vi "svx_Timebase Exec Commands.vi"(5 "Display State In":T2={"X Scale"={"Name"="Time", "FString"="%#.2g", "Major Color"=16777238, "Minor Color"=16777216, "Grid Style"=1, "Maximum"=0.5, "Minimum"=0.0, "Autoscale"=TRUE, "Show Scale Label"={"Probe X"=FALSE, "Probe Y"=TRUE}, "Show Scale"={"Probe X"=TRUE, "Probe Y"=TRUE}, "Autoscale Once"=FALSE}, "Y Scale"={"Name"="Amplitude", "FString"="%#.2g", "Major Color"=16777238, "Minor Color"=16777216, "Scale Visible"=TRUE, " Label Visible"=TRUE, "Grid Style"=1, "Autoscale"=TRUE, "Maximum"={"Probe X"=1.0, "Probe Y"=1.0}, "Minimum"={"Probe X"=-1.0, "Probe Y"=-1.0}, "Autoscale Once"=FALSE}, "Plot"={"Point Style"=0, "Line Width"=0, "Line Style"=0, "Plot Color"=16860, "Point/fill"=16860}, "Tacho Point Color"=16711680, "Property Name"=[], "Container Bounds"={"Width"=640, "Height"=360}, "Background color"=16777226, "Legend Visible"=TRUE, "Scale Range Change"=refnum, "Strings[]"={"Custom pair name"=FALSE, "Row Strings []"=[], "Column Strings []"=[]}, "Cursor"={"Cursor Point Style"=13, "Cursor Style"=5, "Cursor Line Width"=1, "Cursor Line Style"=0, "Cursor Color"=16860, "Cursor Name Visible"=TRUE, "Cursor Visible"=TRUE, "Cursor Lock"=FALSE, "Cursor Index"=0}, "Index"=[], "Legend Width"=200, " Parents Tags"=[], "Children Tags"=[], "Open?"=[], "Label"="Timebase Plot", "Cursor X Pos"={"X"=0.0, "Y"=0.0}, "Cursor Y Pos"={"X"=0.0, "Y"=0.0}, "Graph Type"=enum."Probe X and Y", "Prev Graph Type"=enum."Probe X and Y", "Prev Legend Visible"=TRUE, "Cursor Release"=refnum, "Pair Strings Changed?"=FALSE, "Cursor ID"=refnum, "Legend Background"=16777226, "Legend Font"=16777222, "Probe Y Label"="Probe Y", "Probe X Label"="Probe X", "Probe X Label Visible"=TRUE, "Probe Y Label Visible"=TRUE, "Tree Item Width"=200, "# Custom RowStr"=0, "# Custom ColStr"=0, "Property Name"=refnum, "Data Related State"=refnum} caption="State", 7 "Data In":T7, 8 "Commands":T6[](array[typedef]), 9 "Facade VI":refnum<vi>, 10 "Ref Ins":T1, 11 "Container":refnum<vi>) -> (3 "Display State Out":T2={"X Scale"={"Name"="Time", "FString"="%#.2g", "Major Color"=16777238, "Minor Color"=16777216, "Grid Style"=1, "Maximum"=0.5, "Minimum"=0.0, "Autoscale"=TRUE, "Show Scale Label"={"Probe X"=FALSE, "Probe Y"=TRUE}, "Show Scale"={"Probe X"=TRUE, "Probe Y"=TRUE}, "Autoscale Once"=FALSE}, "Y Scale"={"Name"="Amplitude", "FString"="%#.2g", "Major Color"=16777238, "Minor Color"=16777216, "Scale Visible"=TRUE, " Label Visible"=TRUE, "Grid Style"=1, "Autoscale"=TRUE, "Maximum"={"Probe X"=1.0, "Probe Y"=1.0}, "Minimum"={"Probe X"=-1.0, "Probe Y"=-1.0}, "Autoscale Once"=FALSE}, "Plot"={"Point Style"=0, "Line Width"=0, "Line Style"=0, "Plot Color"=16860, "Point/fill"=16860}, "Tacho Point Color"=16711680, "Property Name"=[], "Container Bounds"={"Width"=640, "Height"=360}, "Background color"=16777226, "Legend Visible"=TRUE, "Scale Range Change"=refnum, "Strings[]"={"Custom pair name"=FALSE, "Row Strings []"=[], "Column Strings []"=[]}, "Cursor"={"Cursor Point Style"=13, "Cursor Style"=5, "Cursor Line Width"=1, "Cursor Line Style"=0, "Cursor Color"=16860, "Cursor Name Visible"=TRUE, "Cursor Visible"=TRUE, "Cursor Lock"=FALSE, "Cursor Index"=0}, "Index"=[], "Legend Width"=200, " Parents Tags"=[], "Children Tags"=[], "Open?"=[], "Label"="Timebase Plot", "Cursor X Pos"={"X"=0.0, "Y"=0.0}, "Cursor Y Pos"={"X"=0.0, "Y"=0.0}, "Graph Type"=enum."Probe X and Y", "Prev Graph Type"=enum."Probe X and Y", "Prev Legend Visible"=TRUE, "Cursor Release"=refnum, "Pair Strings Changed?"=FALSE, "Cursor ID"=refnum, "Legend Background"=16777226, "Legend Font"=16777222, "Probe Y Label"="Probe Y", "Probe X Label"="Probe X", "Probe X Label Visible"=TRUE, "Probe Y Label Visible"=TRUE, "Tree Item Width"=200, "# Custom RowStr"=0, "# Custom ColStr"=0, "Property Name"=refnum, "Data Related State"=refnum} caption="State")   [LabVIEW 2017, in "SVX Timebase.xctl"]
uses:
  <vilib>/addons/_XControls/Timebase Plot/SVX Timebase.xctl
  <vilib>/addons/_XControls/Timebase Plot/subVIs/svx_Timebase Data.ctl
  <vilib>/addons/_XControls/Timebase Plot/subVIs/svx_Timebase State.ctl
  <vilib>/addons/_XControls/Timebase Plot/subVIs/svx_Timebase Bounds.ctl
  <vilib>/addons/_XControls/Timebase Plot/subVIs/svx_Timebase Graph Types.ctl
  <vilib>/addons/_XControls/Timebase Plot/subVIs/svx_Timebase Data Related State.ctl
  <vilib>/addons/_XControls/Timebase Plot/subVIs/svx_Timebase Core States.ctl
panel:
  out "error out":errorcluster
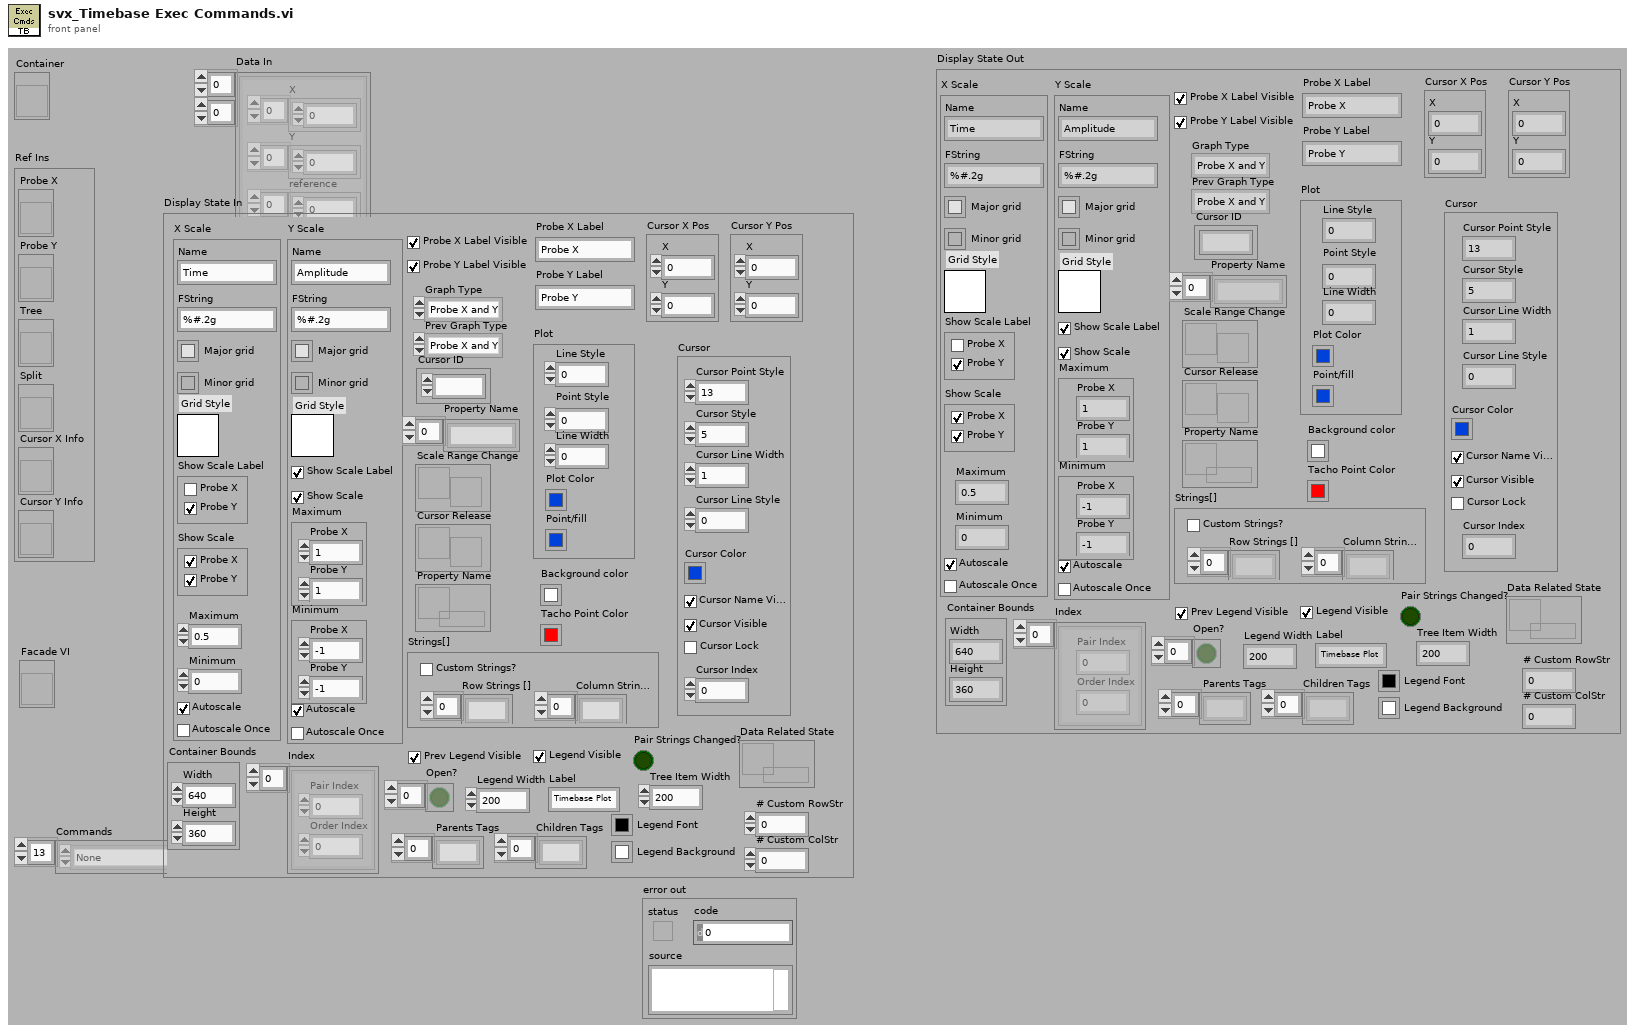
[diagram p1: front panel]
types:
  T1 = cluster{"Probe X":refnum<vi>, "Probe Y":refnum<vi>, "Tree":refnum<vi>, "Split":refnum<vi>, "Cursor X Info":refnum<vi>, "Cursor Y Info":refnum<vi>}
  T2 = typedef "SVX Timebase.xctl/svx_Timebase State.ctl" = cluster{"X Scale":cluster{"Name":string, "FString":string, "Major Color":u32, "Minor Color":u32, "Grid Style":u16, "Maximum":dbl, "Minimum":dbl, "Autoscale":bool, "Show Scale Label":cluster{"Probe X":bool, "Probe Y":bool}, "Show Scale":cluster{"Probe X":bool, "Probe Y":bool}, "Autoscale Once":bool}, "Y Scale":cluster{"Name":string, "FString":string, "Major Color":u32, "Minor Color":u32, "Scale Visible":bool, " Label Visible":bool, "Grid Style":u16, "Autoscale":bool, "Maximum":cluster{"Probe X":dbl, "Probe Y":dbl}, "Minimum":cluster{"Probe X":dbl, "Probe Y":dbl}, "Autoscale Once":bool}, "Plot":cluster{"Point Style":u8, "Line Width":u8, "Line Style":u8, "Plot Color":u32, "Point/fill":u32}, "Tacho Point Color":u32, "Property Name":string[], "Container Bounds":T3, "Background color":u32, "Legend Visible":bool, "Scale Range Change":refnum<user-event>, "Strings[]":cluster{"Custom pair name":bool, "Row Strings []":string[], "Column Strings []":string[]}, "Cursor":cluster{"Cursor Point Style":u8, "Cursor Style":u8, "Cursor Line Width":u8, "Cursor Line Style":u8, "Cursor Color":u32, "Cursor Name Visible":bool, "Cursor Visible":bool, "Cursor Lock":bool, "Cursor Index":i32}, "Index":cluster{"Pair Index":u32, "Order Index":u32}[], "Legend Width":u32, " Parents Tags":string[], "Children Tags":string[], "Open?":bool[], "Label":string, "Cursor X Pos":cluster{"X":dbl, "Y":dbl}, "Cursor Y Pos":cluster{"X":dbl, "Y":dbl}, "Graph Type":T4, "Prev Graph Type":T4, "Prev Legend Visible":bool, "Cursor Release":refnum<user-event>, "Pair Strings Changed?":bool, "Cursor ID":refnum<k1>, "Legend Background":u32, "Legend Font":u32, "Probe Y Label":string, "Probe X Label":string, "Probe X Label Visible":bool, "Probe Y Label Visible":bool, "Tree Item Width":u32, "# Custom RowStr":u32, "# Custom ColStr":u32, "Property Name":refnum<queue>, "Data Related State":T5}
  T3 = typedef "SVX Timebase.xctl/svx_Timebase Bounds.ctl" = cluster{"Width":u32, "Height":u32}
  T4 = typedef "SVX Timebase.xctl/svx_Timebase Graph Types.ctl" = enum16{"Probe X", "Probe Y", "Probe X and Y"}
  T5 = typedef "SVX Timebase.xctl/svx_Timebase Data Related State.ctl" = refnum<queue>
  T6 = typedef "SVX Timebase.xctl/svx_Timebase Core States.ctl" = enum16{"None", "[Axis] Range X Scale", "[Axis] Range Y Scale", "[Layout] Graph Type Change", "[Plot] Tacho Point", "[Plot] Grid and BG", "[Cursor] Cursor Info", "[Legend] Pair Strings", "[Data] Plot Data", "[Legend] Checkbox", "[Layout] Update", "[Legend] Tree Open", "[Layout] Legend Visible Change", "[Plot] Data Point", "[Cursor] Appearance", "[Cursor] Index", "[Legend] Color", "[Axis] Axis and Label", "[Axis] Format String", "[Layout] Min Pane Size", "[Data] Index", "[Plot] Caption", "[Data] Legend Strings"}
  T7 = typedef "SVX Timebase.xctl/svx_Timebase Data.ctl" = cluster{"X":dbl[], "Y":dbl[], "reference":dbl[], "plot type":enum16{"Filtered Plot", "Unfiltered Plot"}, "attribute":variant}[][]
  T8 = cluster{"Queue Newer?":bool, "State Newer?":bool, "Maximum":dbl, "Minimum":dbl, "Maximum":cluster{"Probe X":dbl, "Probe Y":dbl}, "Minimum":cluster{"Probe X":dbl, "Probe Y":dbl}, "Cursor Index":i32, "Cursor X Pos":cluster{"X":dbl, "Y":dbl}, "Cursor Y Pos":cluster{"X":dbl, "Y":dbl}, "Strings[]":cluster{"Custom pair name":bool, "Row Strings []":string[], "Column Strings []":string[]}, "Index":cluster{"Pair Index":u32, "Order Index":u32}[], "Tree Item Width":u32, "Parents Tags":string[], "Children Tags":string[], "Open?":bool[], "Tree Visible?":bool, "Graph Type":T4, "Container Bounds":T3, "Label":string}
  T9 = cluster{"X":dbl[], "Y":dbl[], "reference":dbl[], "plot type":enum16{"Filtered Plot", "Unfiltered Plot"}, "attribute":variant}
  T10 = cluster{"Cursor Point Style":u8, "Cursor Style":u8, "Cursor Line Width":u8, "Cursor Line Style":u8, "Cursor Color":u32, "Cursor Name Visible":bool, "Cursor Visible":bool, "Cursor Lock":bool, "Cursor Index":i32}
  T11 = typedef "LVPointDoubleTypeDef.ctl" = cluster{"Cursor X":dbl, "Cursor Y":dbl}
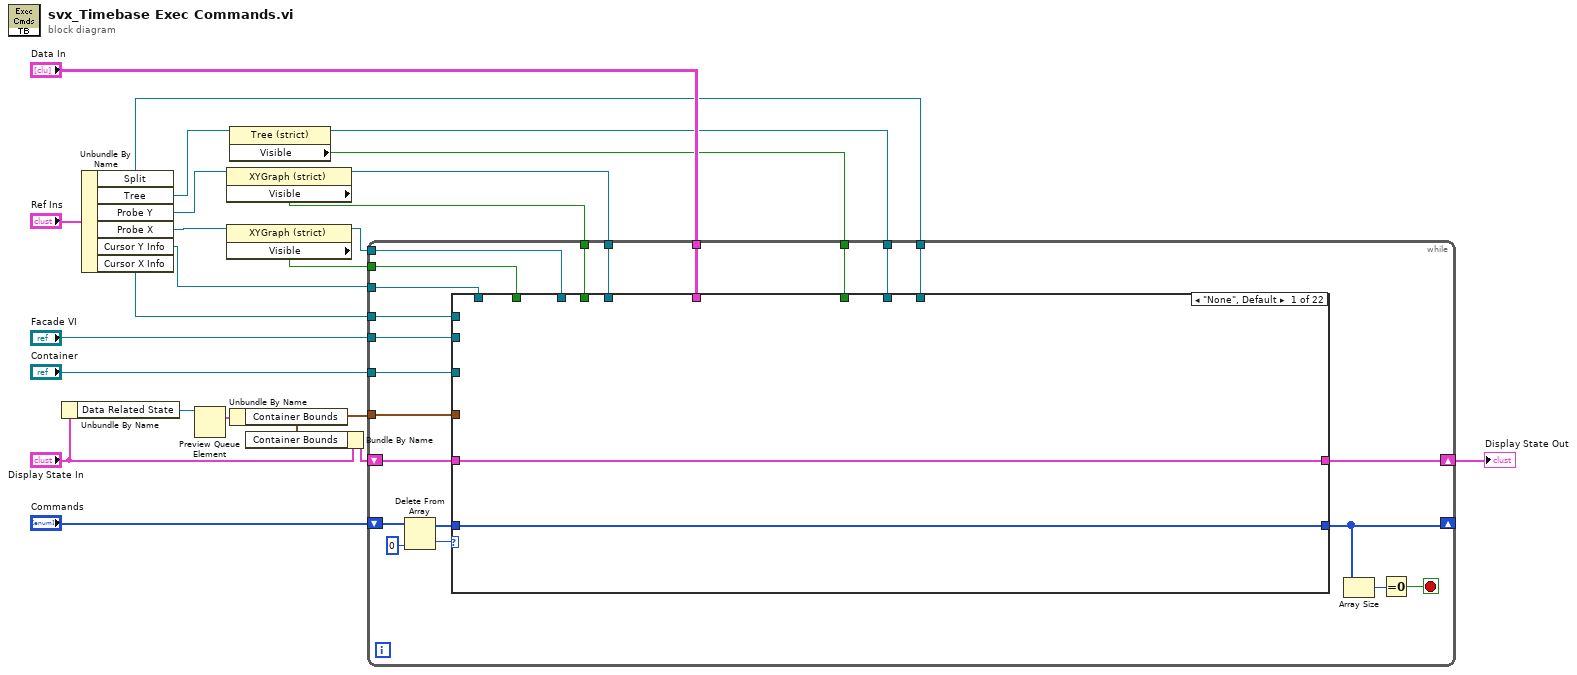
[diagram p0: block diagram]
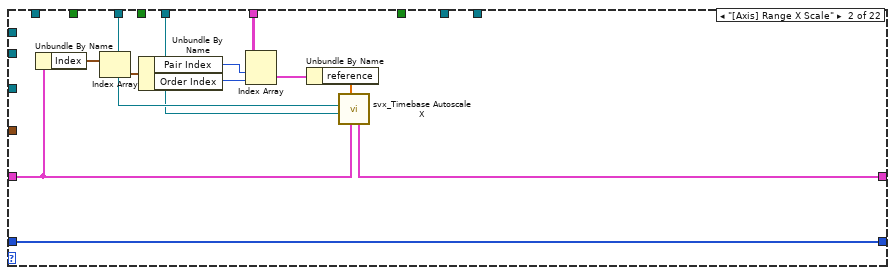
[diagram p2: hidden frame]
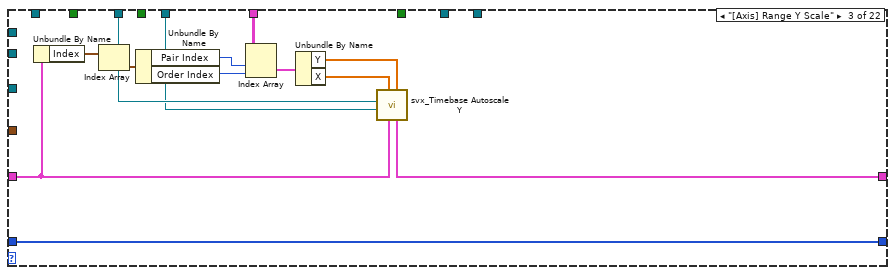
[diagram p3: hidden frame]
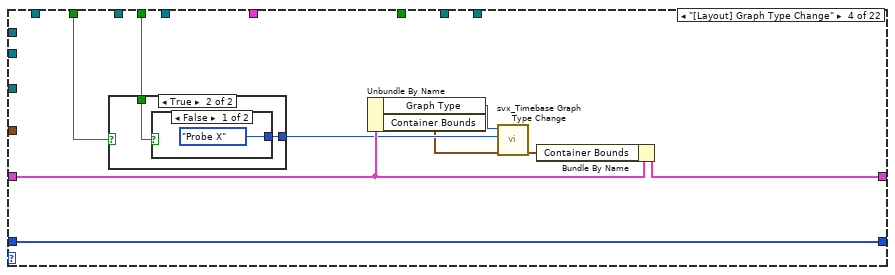
[diagram p4: hidden frame]
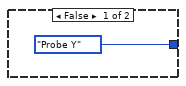
[diagram p5: hidden frame]
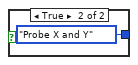
[diagram p6: hidden frame]
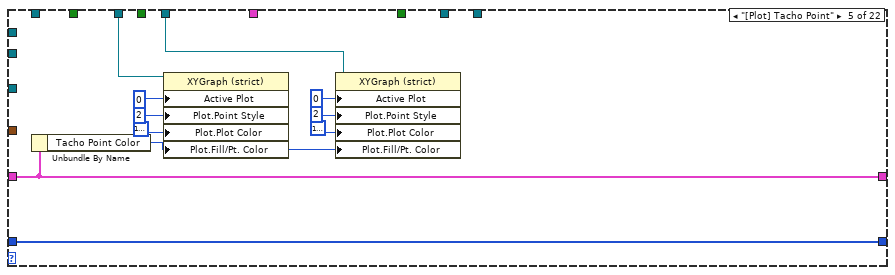
[diagram p7: hidden frame]
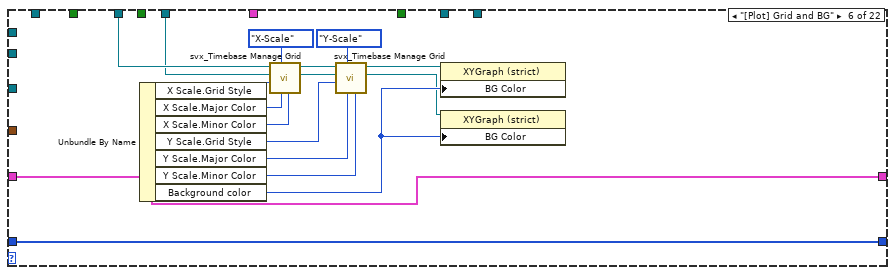
[diagram p8: hidden frame]
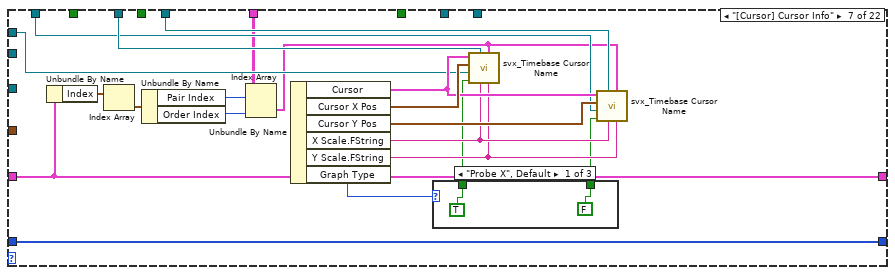
[diagram p9: hidden frame]
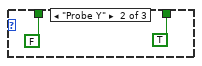
[diagram p10: hidden frame]
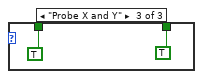
[diagram p11: hidden frame]
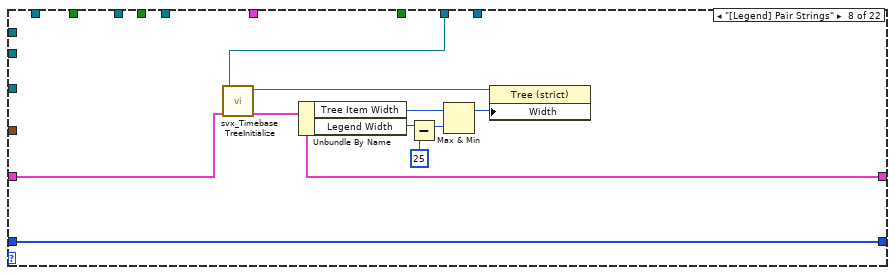
[diagram p12: hidden frame]
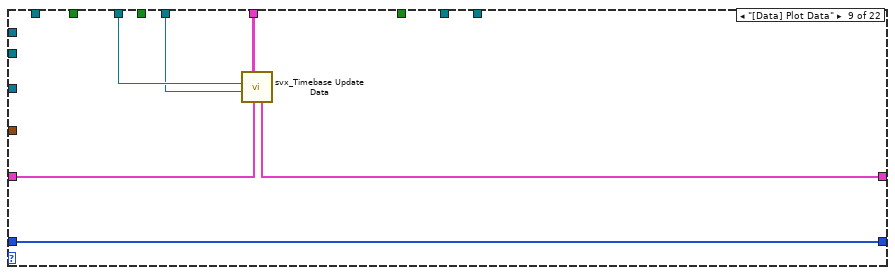
[diagram p13: hidden frame]
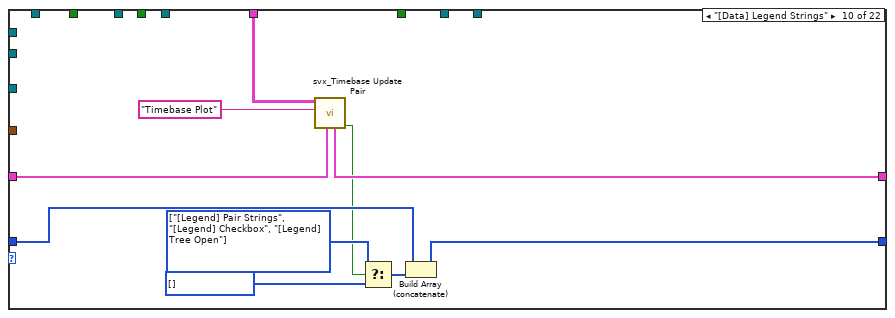
[diagram p14: hidden frame]
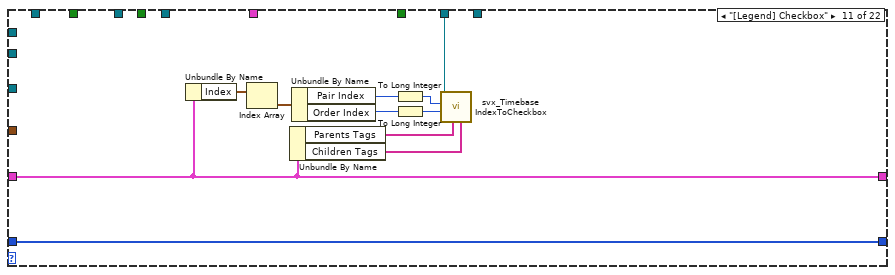
[diagram p15: hidden frame]
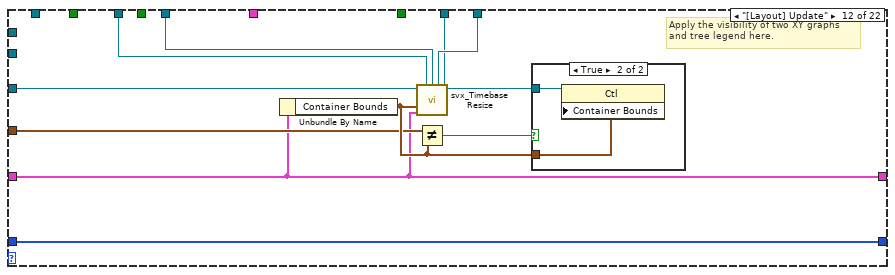
[diagram p16: hidden frame]
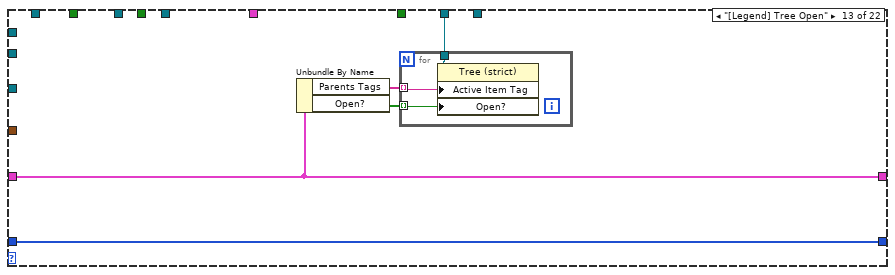
[diagram p18: hidden frame]
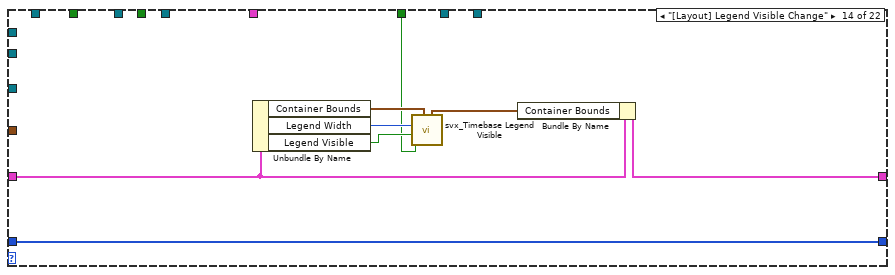
[diagram p19: hidden frame]
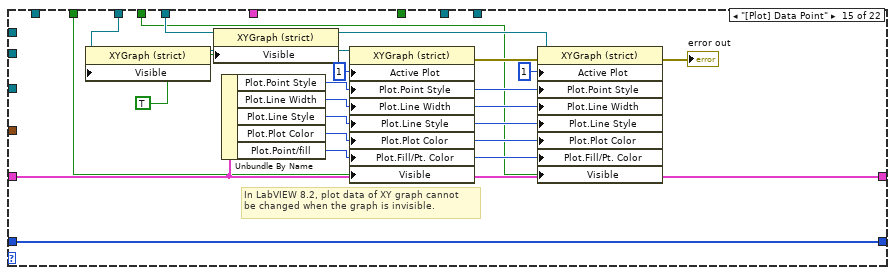
[diagram p20: hidden frame]
diagram:
  n1 = Unbundle By Name("Display State In") -> ("Data Related State"=w2:T5)
  n2 = Unbundle By Name("Ref Ins") -> ("Split"=w7:refnum<vi>, "Tree"=w14:refnum<vi>, "Probe Y"=w17:refnum<vi>, "Probe X"=w18:refnum<vi>, "Cursor Y Info"=w12:refnum<vi>, "Cursor X Info"=w11:refnum<vi>)
  n3 = Preview Queue Element(queue=w2) -> (element=w1:T8)  [unwired: 2 in, 3 out]
  n4 = property class="XYGraph (strict)"(reference=w17) -> (reference out=w4:refnum<vi>, "Visible"=w15:bool)  [unwired: 1 in, 1 out]
  n5 = property class="XYGraph (strict)"(reference=w18) -> (reference out=w5:refnum<vi>, "Visible"=w16:bool)  [unwired: 1 in, 1 out]
  n6 = property class="Tree (strict)"(reference=w14) -> (reference out=w3:refnum<vi>, "Visible"=w13:bool)  [unwired: 1 in, 1 out]
  n7 = Unbundle By Name(w1) -> ("Container Bounds"=w19:T3)
  n8 = Bundle By Name(cluster="Display State In", "Container Bounds"=w19) -> (w20:T2)
  n9 = while {
    shift-right: [w44] -> w6
    shift-left: w20 -> [w45]
    tunnel: w5 -> [w26]
    tunnel: w4 -> [w25]
    tunnel: "Container" -> [w31]
    tunnel: "Data In" -> [w43]
    tunnel: w3 -> [w24]
    tunnel: w7 -> [w42]
    tunnel: w11 -> [w41]
    tunnel: w12 -> [w40]
    shift-right: [w32] -> _
    shift-left: "Commands" -> [w39]
    tunnel: "Facade VI" -> [w33]
    tunnel: w19 -> [w30]
    tunnel: w16 -> [w29]
    tunnel: w15 -> [w28]
    tunnel: w13 -> [w27]
    stop <- w34 stop-if-true
    n10 = Delete From Array(array=w39, index=0) -> (deleted portion=w38:T6, array with subset deleted=w36:T6[])  [unwired: 1 in]
    n11 = case shown="\"None\", Default" w38 {
      tunnel: w45 -> [w47 w54 w62 w81 w97 w112 w115 w148 w154 w161 w169 w179 w192 w201 w220 w225 w233 w242 w271 w274 w286 w297]
      tunnel: [w47 w57 w72 w80 w97 w112 w115 w147 w153 w160 w169 w179 w192 w200 w220 w225 w233 w243 w271 w274 w286 w297] -> w44
      tunnel: w43 -> [_ w51 w61 _ _ _ w114 _ w152 w162 _ _ _ _ _ _ _ _ _ _ _ _]
      tunnel: w25 -> [_ w58 w68 _ w88 w100 w132 _ w150 _ _ w177 _ _ w207 w223 w232 w245 _ w279 w287 _]
      tunnel: w26 -> [_ w59 w69 _ w89 w102 w128 _ w151 _ _ w178 _ _ w209 w224 w231 w252 _ w280 w288 _]
      tunnel: w24 -> [_ _ _ _ _ _ _ w145 _ _ w173 w176 w188 _ _ _ _ _ w268 _ _ _]
      tunnel: w42 -> [_ _ _ _ _ _ _ _ _ _ _ w184 _ _ _ _ _ _ _ _ _ _]
      tunnel: w41 -> [_ _ _ _ _ _ w125 _ _ _ _ _ _ _ _ _ _ _ _ _ _ _]
      tunnel: w40 -> [_ _ _ _ _ _ w124 _ _ _ _ _ _ _ _ _ _ _ _ _ _ _]
      tunnel: w36 -> [w46 w56 w67 w79 w87 w99 w123 w144 w149 w158 w172 w185 w189 w203 w221 w222 w230 w251 w267 w273 w285 w296]
      tunnel: [w46 w56 w67 w79 w87 w99 w123 w144 w149 w157 w172 w185 w189 w203 w221 w222 w230 w251 w267 w273 w285 w296] -> w32
      tunnel: w33 -> [_ _ _ _ _ _ _ _ _ _ _ _ _ _ _ _ _ _ _ _ _ w292]
      tunnel: w31 -> [_ _ _ _ _ _ _ _ _ _ _ w182 _ _ _ _ _ _ _ _ _ _]
      tunnel: w30 -> [_ _ _ _ _ _ _ _ _ _ _ w180 _ _ _ _ _ _ _ _ _ _]
      tunnel: w29 -> [_ _ _ w74 _ _ _ _ _ _ _ _ _ _ w204 _ _ _ _ _ _ _]
      tunnel: w28 -> [_ _ _ w73 _ _ _ _ _ _ _ _ _ _ w205 _ _ _ _ _ _ _]
      tunnel: w27 -> [_ _ _ _ _ _ _ _ _ _ _ _ _ w197 _ _ _ _ _ _ _ _]
      frame "None", Default {
      }
      frame "[Axis] Range X Scale" {
        n12 = Unbundle By Name(w54) -> ("Index"=w53:cluster{"Pair Index":u32, "Order Index":u32}[])
        n13 = Index Array(array=w53) -> (element=w52:cluster{"Pair Index":u32, "Order Index":u32})  [unwired: 1 in]
        n14 = Unbundle By Name(w52) -> ("Pair Index"=w50:u32, "Order Index"=w49:u32)
        n15 = Index Array(array=w51, index (row)=w50, index (col)=w49) -> (element=w48:T9)
        n16 = Unbundle By Name(w48) -> ("reference"=w55:dbl[])
        n17 = call <vilib>:"svx_Timebase Autoscale X.vi"("State In"=w54, "Time Ref"=w55, "Probe Y"=w58, "Probe X"=w59) -> ("State Out"=w57:T2)  [unwired: 7 in]
      }
      frame "[Axis] Range Y Scale" {
        n18 = Unbundle By Name(w62) -> ("Index"=w64:cluster{"Pair Index":u32, "Order Index":u32}[])
        n19 = Index Array(array=w64) -> (element=w65:cluster{"Pair Index":u32, "Order Index":u32})  [unwired: 1 in]
        n20 = Unbundle By Name(w65) -> ("Pair Index"=w63:u32, "Order Index"=w66:u32)
        n21 = Index Array(array=w61, index (row)=w63, index (col)=w66) -> (element=w60:T9)
        n22 = Unbundle By Name(w60) -> ("Y"=w71:dbl[], "X"=w70:dbl[])
        n23 = call <vilib>:"svx_Timebase Autoscale Y.vi"("Y"=w71, "State In"=w62, "X"=w70, "Probe Y"=w68, "Probe X"=w69) -> ("State Out"=w72:T2)  [unwired: 6 in]
      }
      frame "[Layout] Graph Type Change" {
        n24 = case shown="True" w74 {
          tunnel: w73 -> [_ w84]
          tunnel: [svx_Timebase_Graph_Types."Probe Y" ("Graph Type") w83] -> w77
          frame False {
          }
          frame True {
            n25 = case shown="False" w84 {
              tunnel: [svx_Timebase_Graph_Types."Probe X" ("Graph Type") svx_Timebase_Graph_Types."Probe X and Y" ("Graph Type")] -> w83
              frame False {
              }
              frame True {
              }
            }
          }
        }
        n26 = Unbundle By Name(w81) -> ("Graph Type"=w78:T4, "Container Bounds"=w75:T3)
        n27 = call <vilib>:"svx_Timebase Graph Type Change.vi"("Container Bounds In"=w75, "Prev Graph Type"=w77, "Graph Type"=w78) -> ("Container Bounds Out"=w76:T3)  [unwired: 8 in]
        n28 = Bundle By Name(cluster=w81, "Container Bounds"=w76) -> (w80:T2)
      }
      frame "[Plot] Tacho Point" {
        n29 = Unbundle By Name(w97) -> ("Tacho Point Color"=w90:u32)
        n30 = property on="Property Node" class="XYGraph (strict)"(reference=w89, "Active Plot"=u32 0, "Plot.Point Style"=u8 2, "Plot.Plot Color"=u32 16777216, "Plot.Fill/Pt. Color"=w90) -> ()  [unwired: 1 in, 2 out]
        n31 = property on="Property Node" class="XYGraph (strict)"(reference=w88, "Active Plot"=u32 0, "Plot.Point Style"=u8 2, "Plot.Plot Color"=u32 16777216, "Plot.Fill/Pt. Color"=w90) -> ()  [unwired: 1 in, 2 out]
      }
      frame "[Plot] Grid and BG" {
        n32 = Unbundle By Name(w112) -> ("X Scale.Grid Style"=w111:u16, "X Scale.Major Color"=w109:u32, "X Scale.Minor Color"=w98:u32, "Y Scale.Grid Style"=w106:u16, "Y Scale.Major Color"=w105:u32, "Y Scale.Minor Color"=w104:u32, "Background color"=w101:u32)
        n33 = call <vilib>:"svx_Timebase Manage Grid.vi"("Minor Color"=w98, "Major Color"=w109, "Axis"=enum16{"X-Scale", "Y-Scale", "Z-Scale"}."X-Scale", "Grid Style"=w111, "Probe Y in"=w100, "Probe X in"=w102) -> ("Probe Y out"=w107:refnum<vi>, "Probe X out"=w108:refnum<vi>)  [unwired: 2 in, 2 out]
        n34 = call <vilib>:"svx_Timebase Manage Grid.vi"("Minor Color"=w104, "Major Color"=w105, "Axis"=enum16{"X-Scale", "Y-Scale", "Z-Scale"}."Y-Scale", "Grid Style"=w106, "Probe Y in"=w107, "Probe X in"=w108) -> ()  [unwired: 2 in, 4 out]
        n35 = property class="XYGraph (strict)"(reference=w102, "BG Color"=w101) -> ()  [unwired: 1 in, 2 out]
        n36 = property class="XYGraph (strict)"(reference=w100, "BG Color"=w101) -> ()  [unwired: 1 in, 2 out]
      }
      frame "[Cursor] Cursor Info" {
        n37 = Unbundle By Name(w115) -> ("Index"=w117:cluster{"Pair Index":u32, "Order Index":u32}[])
        n38 = Index Array(array=w117) -> (element=w118:cluster{"Pair Index":u32, "Order Index":u32})  [unwired: 1 in]
        n39 = Unbundle By Name(w118) -> ("Pair Index"=w116:u32, "Order Index"=w119:u32)
        n40 = Index Array(array=w114, index (row)=w116, index (col)=w119) -> (element=w113:T9)
        n41 = Unbundle By Name(w115) -> ("Cursor"=w129:T10, "Cursor X Pos"=w131:cluster{"X":dbl, "Y":dbl}, "Cursor Y Pos"=w130:cluster{"X":dbl, "Y":dbl}, "X Scale.FString"=w127:string, "Y Scale.FString"=w126:string, "Graph Type"=w122:T4)
        n42 = case shown="\"Probe X\", Default" w122 {
          tunnel: [TRUE FALSE TRUE] -> w121
          tunnel: [FALSE TRUE TRUE] -> w120
          frame "Probe X", Default {
          }
          frame "Probe Y" {
          }
          frame "Probe X and Y" {
          }
        }
        n43 = call <vilib>:"svx_Timebase Cursor Name.vi"("Y FString"=w126, "Data"=w113, "X FString"=w127, "Probe Ref"=w128, "Subplot Visible?"=w121, "Cursor Info"=w125, "Cursor Position"=w131, "Cursor"=w129) -> ()  [unwired: 4 in]
        n44 = call <vilib>:"svx_Timebase Cursor Name.vi"("Y FString"=w126, "Data"=w113, "X FString"=w127, "Probe Ref"=w132, "Subplot Visible?"=w120, "Cursor Info"=w124, "Cursor Position"=w130, "Cursor"=w129) -> ()  [unwired: 4 in]
      }
      frame "[Legend] Pair Strings" {
        n45 = call <vilib>:"svx_Timebase TreeInitialize.vi"("State in"=w148, "Tree ref in"=w145) -> ("State out"=w147:T2, "Tree ref out"=w146:refnum<vi>)  [unwired: 8 in]
        n46 = Unbundle By Name(w147) -> ("Tree Item Width"=w140:u32, "Legend Width"=w142:u32)
        n47 = Subtract(x=w142, y=u32 25) -> (x-y=w141:u32)
        n48 = Max & Min(x=w140, y=w141) -> (max(x,y)=w139:u32)  [unwired: 1 out]
        n49 = property class="Tree (strict)"(reference=w146, "Width"=w139) -> ()  [unwired: 1 in, 2 out]
      }
      frame "[Data] Plot Data" {
        n50 = call <vilib>:"svx_Timebase Update Data.vi"("State in"=w154, "Data"=w152, "Probe Y"=w150, "Probe X"=w151) -> ("State out"=w153:T2)  [unwired: 7 in]
      }
      frame "[Data] Legend Strings" {
        w163 = T6[] [] items=["None", "[Axis] Range X Scale", "[Axis] Range Y Scale", "[Layout] Graph Type Change", "[Plot] Tacho Point", "[Plot] Grid and BG", "[Cursor] Cursor Info", "[Legend] Pair Strings", "[Data] Plot Data", "[Legend] Checkbox", "[Layout] Update", "[Legend] Tree Open", "[Layout] Legend Visible Change", "[Plot] Data Point", "[Cursor] Appearance", "[Cursor] Index", "[Legend] Color", "[Axis] Axis and Label", "[Axis] Format String", "[Layout] Min Pane Size", "[Data] Index", "[Plot] Caption", "[Data] Legend Strings"]
        w159 = T6[] [enum."[Legend] Pair Strings", enum."[Legend] Checkbox", enum."[Legend] Tree Open"] items=["None", "[Axis] Range X Scale", "[Axis] Range Y Scale", "[Layout] Graph Type Change", "[Plot] Tacho Point", "[Plot] Grid and BG", "[Cursor] Cursor Info", "[Legend] Pair Strings", "[Data] Plot Data", "[Legend] Checkbox", "[Layout] Update", "[Legend] Tree Open", "[Layout] Legend Visible Change", "[Plot] Data Point", "[Cursor] Appearance", "[Cursor] Index", "[Legend] Color", "[Axis] Axis and Label", "[Axis] Format String", "[Layout] Min Pane Size", "[Data] Index", "[Plot] Caption", "[Data] Legend Strings"]
        n51 = call <vilib>:"svx_Timebase Update Pair.vi"("State in"=w161, "Label Text"="Timebase Plot", "timebase plot"=w162) -> ("update tree?"=w156:bool, "State out"=w160:T2)  [unwired: 7 in]
        n52 = Select(t=w159, s=w156, f=w163) -> (s? t:f=w164:T6[])
        n53 = Build Array (concatenate)(w158, w164) -> (w157:T6[])
      }
      frame "[Legend] Checkbox" {
        n54 = Unbundle By Name(w169) -> ("Index"=w170:cluster{"Pair Index":u32, "Order Index":u32}[])
        n55 = Index Array(array=w170) -> (element=w171:cluster{"Pair Index":u32, "Order Index":u32})  [unwired: 1 in]
        n56 = Unbundle By Name(w169) -> ("Parents Tags"=w175:string[], "Children Tags"=w174:string[])
        n57 = Unbundle By Name(w171) -> ("Pair Index"=w168:u32, "Order Index"=w166:u32)
        n58 = To Long Integer(number=w168) -> (32bit integer=w167:i32)
        n59 = To Long Integer(number=w166) -> (32bit integer=w165:i32)
        n60 = call <vilib>:"svx_Timebase IndexToCheckbox.vi"("All Children Tags"=w174, "All parents Tags"=w175, "ColumnIdx"=w165, "RowIdx"=w167, "Tree ref in"=w173) -> ()  [unwired: 6 in, 1 out]
      }
      frame "[Layout] Update" {
        # "Apply the visibility of two XY graphs\nand tree legend here."
        n61 = Unbundle By Name(w179) -> ("Container Bounds"=w181:T3)
        n62 = call <vilib>:"svx_Timebase Resize.vi"("Probe X"=w178, "Probe Y"=w177, "Split"=w184, "Tree"=w176, "Bounds In"=w181, "State In"=w179) -> ()  [unwired: 10 in]
        n63 = Not Equal?(x=w180, y=w181) -> (x != y?=w183:bool)
        n64 = case shown="True" w183 {
          tunnel: w182 -> [_ w187]
          tunnel: w181 -> [_ w186]
          frame False {
          }
          frame True {
            n65 = property class="Ctl"(reference=w187, "Container Bounds"=w186) -> ()  [unwired: 1 in, 2 out]
          }
        }
      }
      frame "[Legend] Tree Open" {
        n66 = Unbundle By Name(w192) -> ("Parents Tags"=w191:string[], "Open?"=w190:bool[])
        n67 = for {
          tunnel: w191 -> [w195] mode=indexing
          tunnel: w190 -> [w194] mode=indexing
          tunnel: w188 -> [w193]
          n68 = property on="Property Node" class="Tree (strict)"(reference=w193, "Active Item Tag"=w195, "Open?"=w194) -> ()  [unwired: 1 in, 2 out]
        }
      }
      frame "[Layout] Legend Visible Change" {
        n69 = Unbundle By Name(w201) -> ("Container Bounds"=w198:T3, "Legend Width"=w199:u32, "Legend Visible"=w202:bool)
        n70 = call <vilib>:"svx_Timebase Legend Visible.vi"("Bounds In"=w198, "Prev Legend Visible"=w197, "Legend Visible"=w202, "Legend Width"=w199) -> ("Bounds Out"=w196:T3)  [unwired: 7 in]
        n71 = Bundle By Name(cluster=w201, "Container Bounds"=w196) -> (w200:T2)
      }
      frame "[Plot] Data Point" {
        w206 = TRUE ("Visible")
        # "In LabVIEW 8.2, plot data of XY graph cannot\nbe changed when the graph is invisible."
        n72 = property class="XYGraph (strict)"(reference=w209, "Visible"=w206) -> (reference out=w210:refnum<vi>)  [unwired: 1 in, 1 out]
        n73 = property class="XYGraph (strict)"(reference=w207, "Visible"=w206) -> (reference out=w208:refnum<vi>)  [unwired: 1 in, 1 out]
        n74 = Unbundle By Name(w220) -> ("Plot.Point Style"=w219:u8, "Plot.Line Width"=w218:u8, "Plot.Line Style"=w217:u8, "Plot.Plot Color"=w216:u32, "Plot.Point/fill"=w215:u32)
        n75 = property on="Property Node" class="XYGraph (strict)"(reference=w210, "Active Plot"=u32 1, "Plot.Point Style"=w219, "Plot.Line Width"=w218, "Plot.Line Style"=w217, "Plot.Plot Color"=w216, "Plot.Fill/Pt. Color"=w215, "Visible"=w204) -> (error out=w211:errorcluster)  [unwired: 1 in, 1 out]
        n76 = property on="Property Node" class="XYGraph (strict)"(reference=w208, error in=w211, "Active Plot"=u32 1, "Plot.Point Style"=w219, "Plot.Line Width"=w218, "Plot.Line Style"=w217, "Plot.Plot Color"=w216, "Plot.Fill/Pt. Color"=w215, "Visible"=w205) -> (error out=→"error out":errorcluster)  [unwired: 1 out]
      }
      frame "[Plot] Caption" {
        n77 = Unbundle By Name(w225) -> ("Probe X Label Visible"=w229:bool, "Probe X Label"=w228:string, "Probe Y Label Visible"=w226:bool, "Probe Y Label"=w227:string)
        n78 = property on="Property Node" class="XYGraph (strict)"(reference=w224, "Caption.Visible"=w229, "Caption.Text"=w228) -> ()  [unwired: 1 in, 2 out]
        n79 = property on="Property Node" class="XYGraph (strict)"(reference=w223, "Caption.Visible"=w226, "Caption.Text"=w227) -> ()  [unwired: 1 in, 2 out]
      }
      frame "[Cursor] Appearance" {
        w239 = u32 0 ("Active Plot")
        n80 = Unbundle By Name(w233) -> ("Cursor.Cursor Color"=w234:u32, "Cursor.Cursor Point Style"=w235:u8, "Cursor.Cursor Style"=w236:u8, "Cursor.Cursor Line Width"=w237:u8, "Cursor.Cursor Line Style"=w238:u8)
        n81 = property on="Property Node" class="XYGraph (strict)"(reference=w231, "Active Cursor"=w239, "Cursor.Cursor Color"=w234, "Cursor.Cursor Point Style"=w235, "Cursor.Cursor Style"=w236, "Cursor.LineWidth"=w237, "Cursor.LineStyle"=w238) -> ()  [unwired: 1 in, 2 out]
        n82 = property on="Property Node" class="XYGraph (strict)"(reference=w232, "Active Cursor"=w239, "Cursor.Cursor Color"=w234, "Cursor.Cursor Point Style"=w235, "Cursor.Cursor Style"=w236, "Cursor.LineWidth"=w237, "Cursor.LineStyle"=w238) -> ()  [unwired: 1 in, 2 out]
      }
      frame "[Cursor] Index" {
        n83 = Unbundle By Name(w242) -> ("Cursor.Cursor Index"=w247:i32)
        n84 = property on="Property Node" class="XYGraph (strict)"(reference=w252, "Active Cursor"=u32 0 ("Active Plot"), "Cursor.Cursor Index"=w247) -> (reference out=w246:refnum<vi>, "Cursor.Cursor Position"=w244:T11)  [unwired: 1 in, 1 out]
        n85 = Not A Number/Path/Refnum?(number/path/refnum=w244) -> (NaN/Path/Refnum?=w250:cluster{"Cursor X":bool, "Cursor Y":bool})
        n86 = Cluster To Array(cluster=w250) -> (array=w249:bool[])
        n87 = Or Array Elements(Boolean array=w249) -> (logical OR=w248:bool)
        n88 = case shown="True" w248 {
          tunnel: w244 -> [w257 _]
          tunnel: [w257 w263] -> w241
          tunnel: [w256 w262] -> w240
          tunnel: w247 -> [w255 w261]
          tunnel: w246 -> [_ w260]
          tunnel: w245 -> [w254 w259]
          frame False {
            n89 = property on="Property Node" class="XYGraph (strict)"(reference=w254, "Active Cursor"=u32 0, "Cursor.Cursor Index"=w255) -> ("Cursor.Cursor Position"=w256:T11)  [unwired: 1 in, 2 out]
          }
          frame True {
            n90 = Increment(x=w261) -> (x+1=w264:i32)
            n91 = property on="Property Node" class="XYGraph (strict)"(reference=w260, "Active Cursor"=u32 0, "Cursor.Cursor Index"=w264) -> ("Cursor.Cursor Position"=w263:T11)  [unwired: 1 in, 2 out]
            n92 = property on="Property Node" class="XYGraph (strict)"(reference=w259, "Active Cursor"=u32 0, "Cursor.Cursor Index"=w264) -> ("Cursor.Cursor Position"=w262:T11)  [unwired: 1 in, 2 out]
          }
        }
        n93 = Bundle By Name(cluster=w242, "Cursor X Pos"=w241, "Cursor Y Pos"=w240) -> (w243:T2)
      }
      frame "[Legend] Color" {
        w272 = -2 ("Active Cell:Active Column Number")
        n94 = Unbundle By Name(w271) -> ("Legend Background"=w269:u32, "Legend Font"=w270:u32)
        n95 = property on="Property Node" class="Tree (strict)"(reference=w268, "ActiveColNum"=w272, "Active Item Row Number"=w272, "CellBG"=w269, "CellFontColor"=w270) -> ()  [unwired: 1 in, 2 out]
      }
      frame "[Axis] Axis and Label" {
        n96 = Unbundle By Name(w274) -> ("X Scale.Name"=w284:string, "Y Scale.Name"=w283:string, "Y Scale.Scale Visible"=w282:bool, "Y Scale.Label Visible"=w281:bool, "X Scale.Show Scale.Probe X"=w278:bool, "X Scale.Show Scale Label.Probe X"=w277:bool, "X Scale.Show Scale.Probe Y"=w276:bool, "X Scale.Show Scale Label.Probe Y"=w275:bool)
        n97 = property on="Property Node" class="XYGraph (strict)"(reference=w280, "XScale.NameLbl.Text"=w284, "YScale.NameLbl.Text"=w283, "YScale.Visible"=w282, "YScale.NameLbl.Visible"=w281, "XScale.Visible"=w278, "XScale.NameLbl.Visible"=w277) -> ()  [unwired: 1 in, 2 out]
        n98 = property on="Property Node" class="XYGraph (strict)"(reference=w279, "XScale.NameLbl.Text"=w284, "YScale.NameLbl.Text"=w283, "YScale.Visible"=w282, "YScale.NameLbl.Visible"=w281, "XScale.Visible"=w276, "XScale.NameLbl.Visible"=w275) -> ()  [unwired: 1 in, 2 out]
      }
      frame "[Axis] Format String" {
        n99 = Unbundle By Name(w286) -> ("X Scale.FString"=w290:string, "Y Scale.FString"=w289:string)
        n100 = property on="Property Node" class="XYGraph (strict)"(reference=w288, "XScale.FormatString"=w290, "YScale.FormatString"=w289) -> ()  [unwired: 1 in, 2 out]
        n101 = property on="Property Node" class="XYGraph (strict)"(reference=w287, "XScale.FormatString"=w290, "YScale.FormatString"=w289) -> ()  [unwired: 1 in, 2 out]
      }
      frame "[Layout] Min Pane Size" {
        n102 = Unbundle By Name(w297) -> ("Legend Visible"=w295:bool, "Legend Width"=w294:u32, "Graph Type"=w293:T4)
        n103 = To Word Integer(number=w294) -> (16bit integer=w291:i16)
        n104 = call <vilib>:"svx_Timebase Set Minimum Panel Size.vi"("Facade VI"=w292, "Graph Type"=w293, "Legend Width"=w291, "Legend Visible"=w295) -> ()  [unwired: 8 in]
      }
    }
    n105 = Array Size(array=w32) -> (size(s)=w35:i32)
    n106 = Equal To 0?(x=w35) -> (x = 0?=w34:bool)
  }
  "Display State Out" <- w6
